vi "createLinearRamp.vi"(7 "ramp time":dbl, 8 "wait time":dbl, 9 "End Voltage":dbl, 10 "Start Voltage":dbl, 11 "dt":dbl) -> (1 "output waveform":waveform(dbl)(graph))   [LabVIEW 2013]
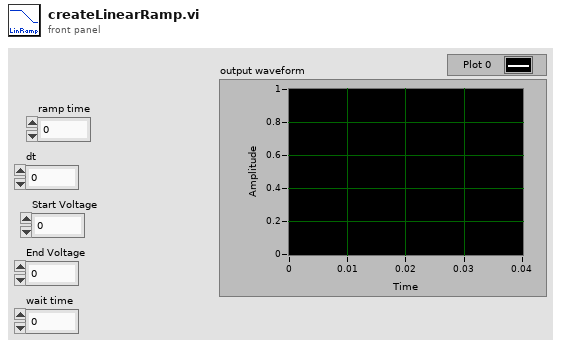
[diagram p1: front panel]
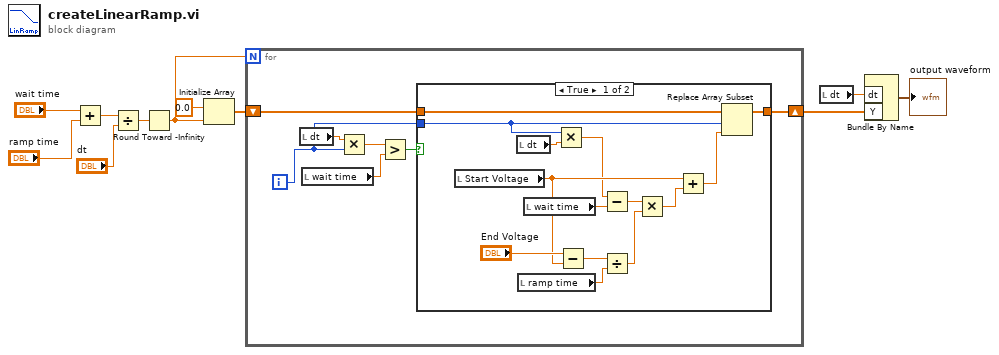
[diagram p0: block diagram]
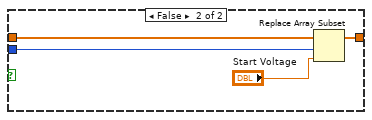
[diagram p2: hidden frame]
diagram:
  n1 = Add(x="wait time", y="ramp time") -> (x+y=w9:dbl)
  n2 = Divide(x=w9, y="dt") -> (x/y=w7:dbl)
  n3 = Round Toward -Infinity(1:w7) -> (0:w4:dbl)
  n4 = Initialize Array(0.0 ("element"), w4) -> (w5:dbl[])
  n5 = for {
    N: w4 -> [_]
    shift-right: [w13] -> w3
    shift-left: w5 -> [w14]
    i -> [w12]
    n6 = local read "dt"() -> (w18:dbl)
    n7 = local read "wait time"() -> (w16:dbl)
    n8 = Multiply(x=w18, y=w12) -> (x*y=w17:dbl)
    n9 = Greater?(x=w17, y=w16) -> (0:w15:bool)
    n10 = case shown="True" w15 {
      tunnel: w14 -> [w32 w36]
      tunnel: [w31 w35] -> w13
      tunnel: w12 -> [w28 w34]
      frame True {
        n11 = local read "Start Voltage"() -> (w22:dbl)
        n12 = local read "dt"() -> (w27:dbl)
        n13 = local read "ramp time"() -> (w29:dbl)
        n14 = local read "wait time"() -> (w20:dbl)
        n15 = Multiply(x=w28, y=w27) -> (x*y=w21:dbl)
        n16 = Subtract(x="End Voltage", y=w22) -> (x-y=w30:dbl)
        n17 = Subtract(x=w21, y=w20) -> (x-y=w19:dbl)
        n18 = Divide(x=w30, y=w29) -> (x/y=w26:dbl)
        n19 = Multiply(x=w19, y=w26) -> (x*y=w25:dbl)
        n20 = Add(x=w22, y=w25) -> (x+y=w24:dbl)
        n21 = Replace Array Subset(array=w32, new element=w24, index=w28) -> (w31:dbl[])
      }
      frame False {
        n22 = Replace Array Subset(array=w36, new element="Start Voltage", index=w34) -> (w35:dbl[])
      }
    }
  }
  n23 = local read "dt"() -> (w2:dbl)
  n24 = Bundle By Name("dt"=w2, "Y"=w3) -> (→"output waveform":waveform(dbl))  [unwired: 1 in]
